vi "TraverseControl.vi"(0 "Mode":T6=enum."Read traverse position", 1 "Work in Tunnel Coordinates?":T3, 2 "Probe Support":T2=[{"Max"=15001.0, "Min"=12000.0}, {"Max"=1000.0, "Min"=-1000.0}, {"Max"=700.0, "Min"=0.0}] {"Min" format="%#.1f"; "Max" format="%#.1f"}, 3 "Model       Roll      Pitch       Yaw (deg)":sgl[](array[numeric]) format="%#.2f", 4 "Probe Volume":T2=[{"Max"=15.0, "Min"=-15.0}, {"Max"=250.0, "Min"=0.0}, {"Max"=15.0, "Min"=-15.0}] {"Min" format="%#.1f"; "Max" format="%#.1f"}, 5 "Position input XYZ":sgl[](array[numeric])=[0.0, 0.0, 0.0] format="%.2f", 6 "Route Checking?":bool, 7 "Entire Space":T2=[{"Max"=15001.0, "Min"=12000.0}, {"Max"=1000.0, "Min"=-1000.0}, {"Max"=700.0, "Min"=0.0}] {"Min" format="%#.1f"; "Max" format="%#.1f"}, 8 "Last Part of Move?":bool, 9 "Home":T1, 10 "Exclude Array":T4[](array[typedef]) {"Sizes"."Min" format="%#.1f"; "Sizes"."Max" format="%#.1f"}, 11 "Speed Factor":sgl=1.0 min=0.1 max=5 format="%.2f", 12 "Traverse Name":string, 13 "Backlash Compensation?":bool=TRUE, 15 "Trav_Coordinates New Pos dx;dy;dz":sgl[](array[numeric])=[0.0, 0.0, 0.0] format="%.2f", 16 "Trav_Coordinates Current Pos dx;dy;dz":sgl[](array[numeric])=[0.0, 0.0, 0.0] format="%.2f") -> (14 "Position Output XYZ":sgl[](array[numeric]) format="%.2f", 17 "Moved?":bool, 18 "Position Correct":bool, 19 "Error String":string)   [LabVIEW 2022 SP3]
uses:
  Anemometry/Anemometry Sub Vis/Gen Trav/Trav_mode.ctl
  Anemometry/Anemometry Sub Vis/Gen Trav/Route mapping/Exclude_cluster.ctl
  Anemometry/Anemometry Sub Vis/Gen Trav/Route mapping/Box_size.ctl
  Anemometry/Anemometry Sub Vis/Gen Trav/Route mapping/Exclusion_type.ctl
  Anemometry/Anemometry Sub Vis/Controls/Tunnel_Coordinates.ctl
  Anemometry/Anemometry Sub Vis/Controls/Home.ctl
  ~subVIs/GenericDriveCommand.ctl
  ADAM Client/Sub VIs/ADAM Controls/Update_scan_value.ctl
  Anemometry/Anemometry Sub Vis/Globals/Preference_global.vi
  Anemometry/Anemometry Sub Vis/Globals/Trav_pos_global.vi
  ~subVIs/DriveConfigGlobal.vi
  ~subVIs/Traverse Type.ctl
panel:
  out "Config the same?":bool[](array[boolean])
  out "Position Steps":sgl[][](array[numeric]) format="%.2f"
  out "Log File":path
  out "Achieved Pos In Eng units of all channels":sgl[](array[numeric]) format="%.2f"
  out "Pulses Positon all channels":sgl[](array[numeric])
  out "Counters Reset?":bool
  # "X                Y                   Z"
  # "X                           Y                          Z"
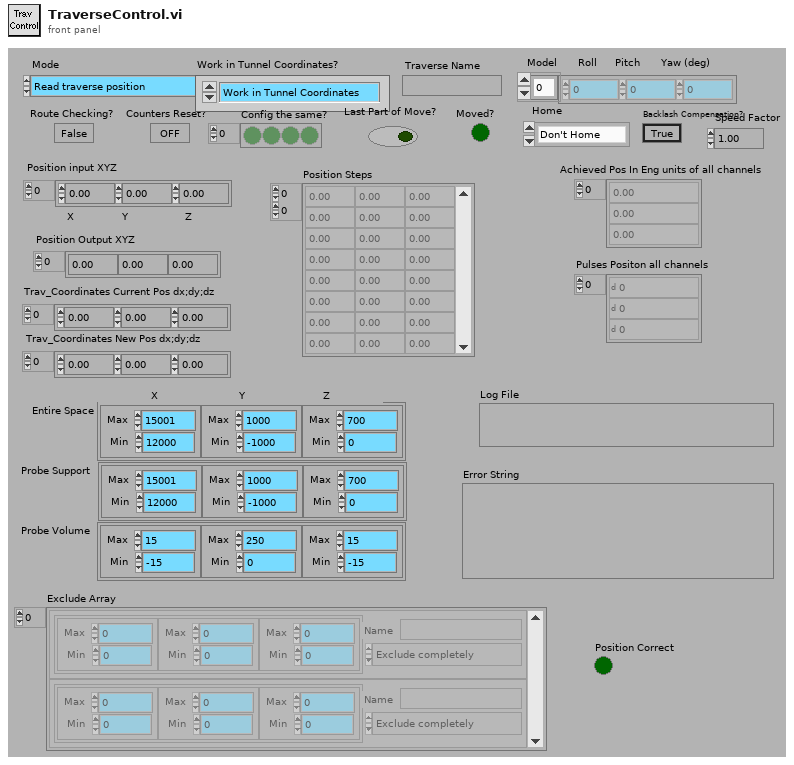
[diagram p1: front panel]
types:
  T1 = typedef "Home.ctl" = enum16{"Don't Home", "Home  +X", "Home  -X", "Home  +Y", "Home  -Y", "Home  +Z", "Home  -Z"}
  T2 = typedef "Box_size.ctl" = cluster{"Max":sgl, "Min":sgl}[]
  T3 = typedef "Tunnel_Coordinates.ctl" = enum16{"Work in Tunnel Coordinates", "Work in Model Coordinates"}
  T4 = typedef "Exclude_cluster.ctl" = cluster{"Sizes":T2, "Name":string, "Exclude Type":T5}
  T5 = typedef "Exclusion_type.ctl" = enum16{"Exclude completely", "Allow only vertical moves"}
  T6 = typedef "Trav_mode.ctl" = enum16{"Move traverse", "Read traverse position", "Teach Position"}
  T7 = typedef "Traverse Type.ctl" = enum16{"MCode", "Dynamixel"}
  T8 = typedef "GenericDriveCommand.ctl" = string
  T9 = enum16{"To Traverse Coordinates", "To User Coordinates"}
  T10 = typedef "DriveProperties.ctl" = cluster{"Channel Name":string, "Vel. Default":sgl, "Acc. Default":sgl, "Vel. Max":sgl, "Vel. Min":sgl, "Acc. Max":sgl, "Acc. Min":sgl, "Pulses/unit":sgl, "Address":u8, "Pulse Offset":i32, "Pos Tolerance":sgl, "Pulses/rev":sgl, "Backlash/Eng units":sgl, "Current Pos":sgl, "Ch Status":enum16{"Active", "Offline", "Simulate"}, "Port Name":string, "Axis Transform mode":string, "Metadata Ch Name":string, "Type":T7, "De Power Motor":enum16{"TRUE", "FALSE"}, "ConfigString":string}
  T11 = typedef "Update_scan_value.ctl" = cluster{"Channel Name":string, "New Value":dbl, "!Auto_Off":bool}
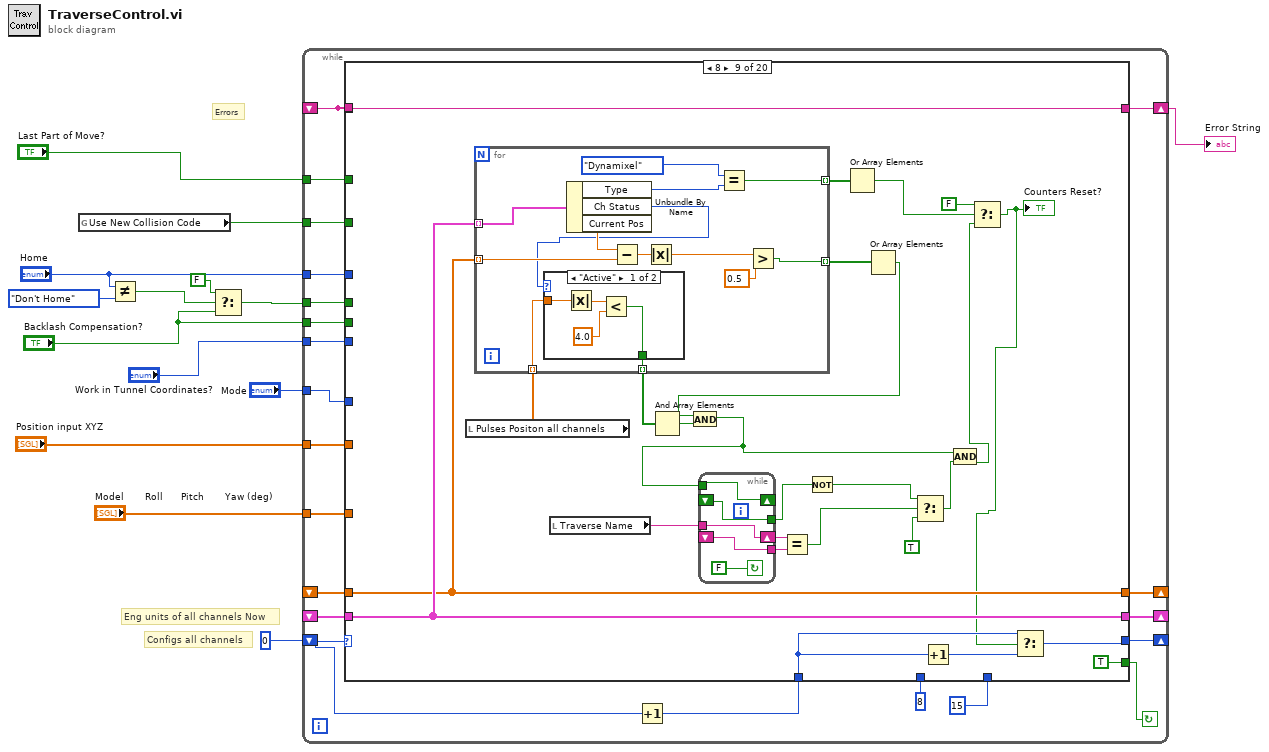
[diagram p0: block diagram]
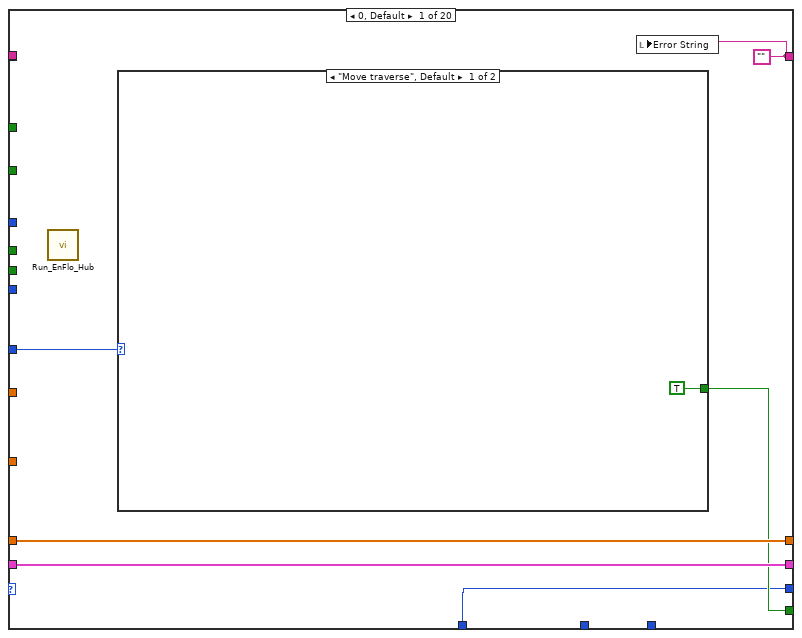
[diagram p2: hidden frame]
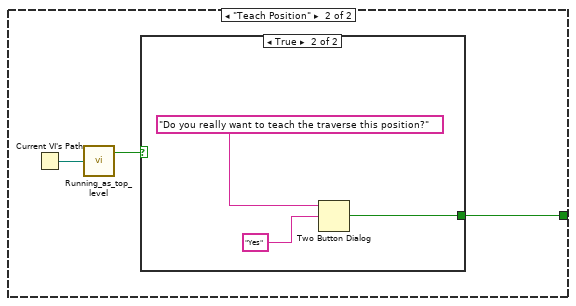
[diagram p3: hidden frame]
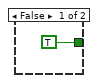
[diagram p4: hidden frame]
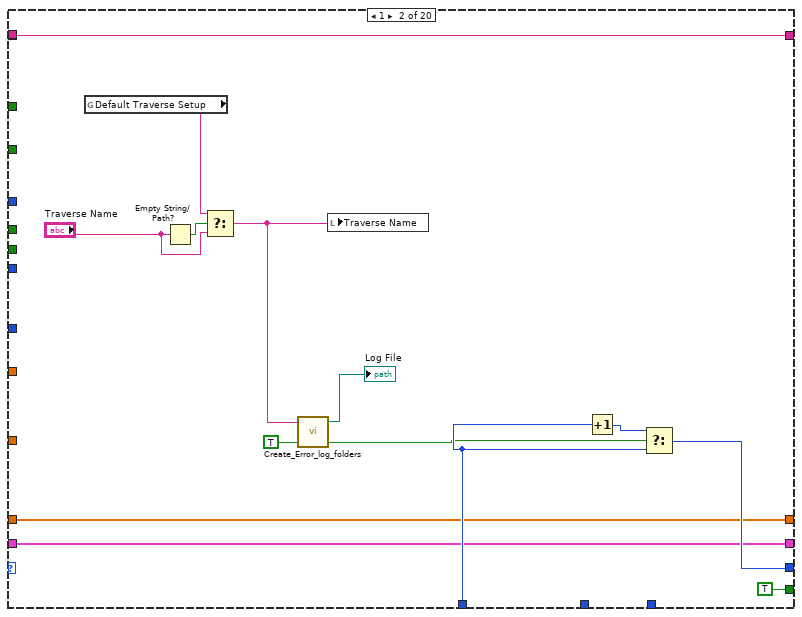
[diagram p5: hidden frame]
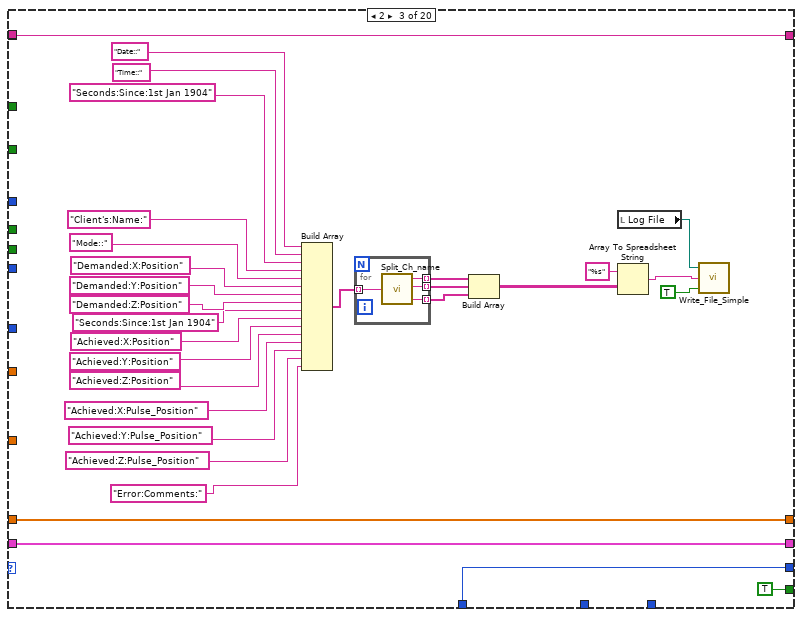
[diagram p6: hidden frame]
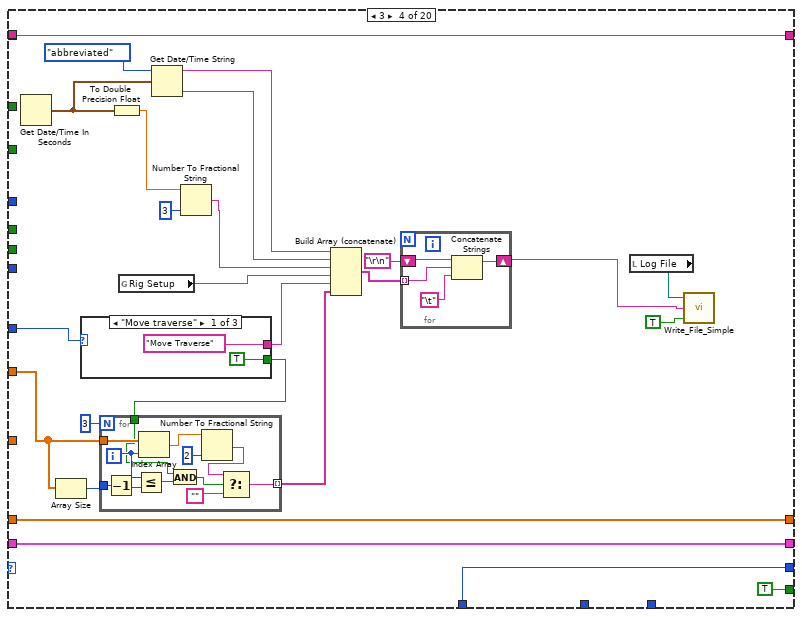
[diagram p7: hidden frame]
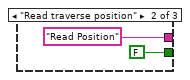
[diagram p8: hidden frame]
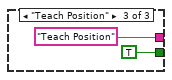
[diagram p9: hidden frame]
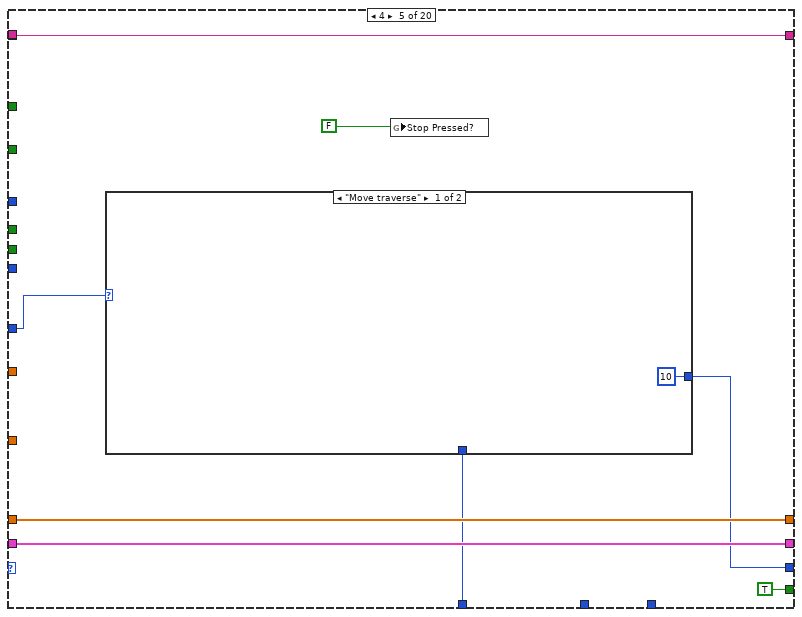
[diagram p10: hidden frame]
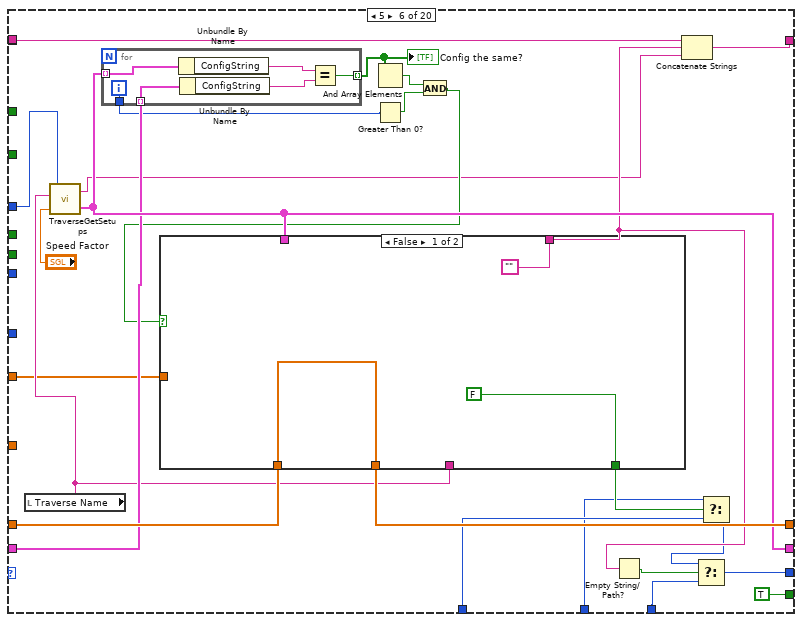
[diagram p12: hidden frame]
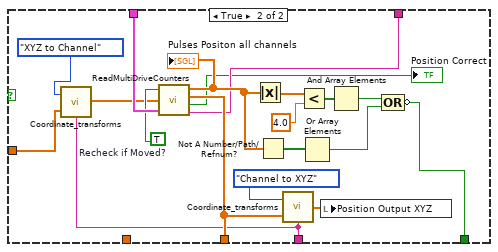
[diagram p13: hidden frame]
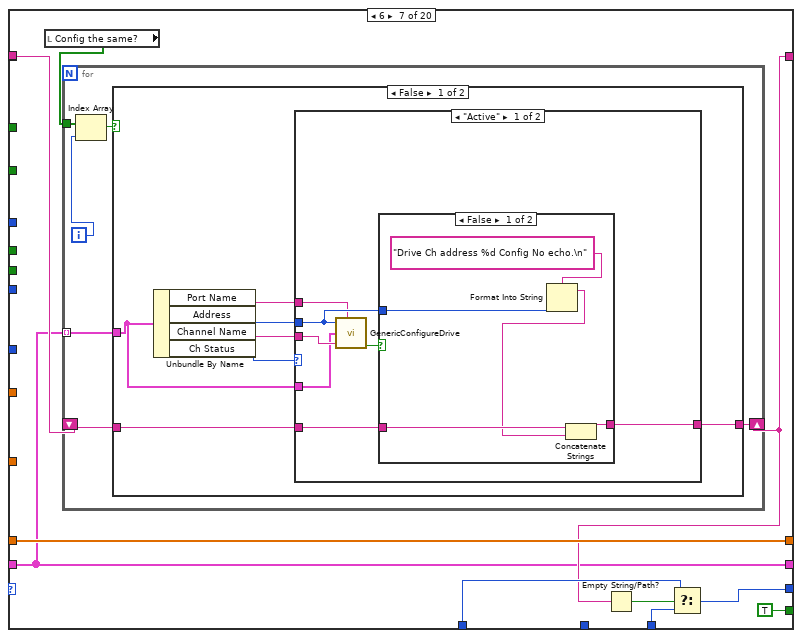
[diagram p14: hidden frame]
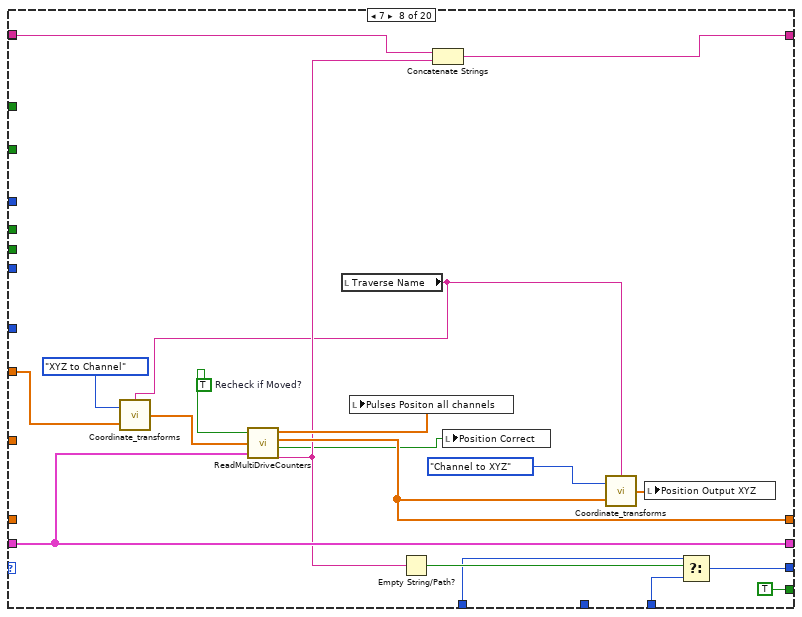
[diagram p18: hidden frame]
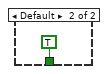
[diagram p19: hidden frame]
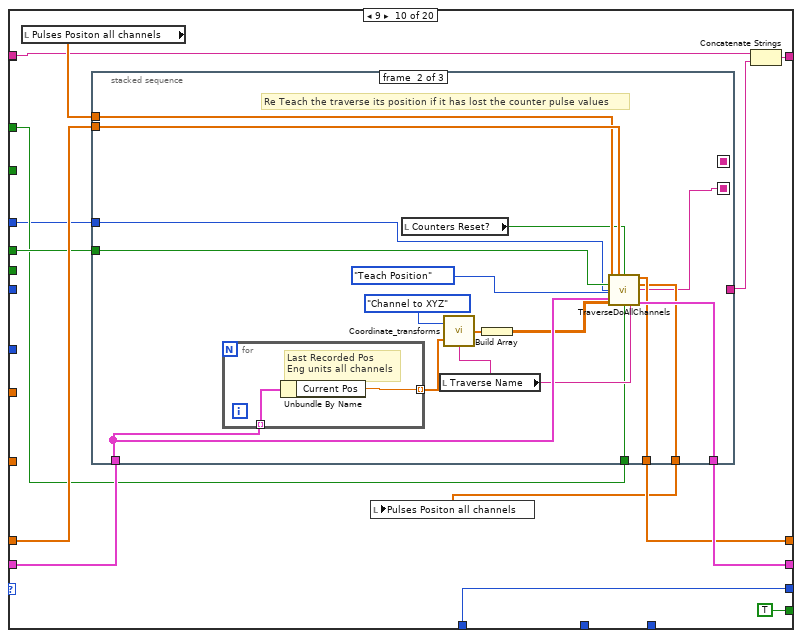
[diagram p20: hidden frame]
diagram:
  # "Errors"
  # "Eng units of all channels Now"
  # "Configs all channels"
  n1 = global read "Preference_global.vi" "Use New Collision Code"() -> (w3:bool)
  n2 = Not Equal?(x="Home", y=Home."Don't Home" ("Home")) -> (x != y?=w4:bool)
  n3 = Select(t=FALSE, s=w4, f="Backlash Compensation?") -> (s? t:f=w8:bool)
  n4 = while {
    tunnel: w8 -> [w22]
    tunnel: "Position input XYZ" -> [w26]
    shift-left: _ -> [w23]
    shift-right: [w27] -> w12
    shift-left: _ -> [w28]
    shift-right: [w29] -> _
    shift-left: _ -> [w17]
    shift-right: [w30] -> _
    shift-left: 0 -> [w33]
    shift-right: [w31] -> _
    tunnel: "Mode" -> [w35]
    tunnel: "Model       Roll      Pitch       Yaw (deg)" -> [w21]
    tunnel: "Work in Tunnel Coordinates?" -> [w20]
    tunnel: "Last Part of Move?" -> [w19]
    tunnel: "Home" -> [w18]
    tunnel: w3 -> [w16]
    tunnel: "Backlash Compensation?" -> [w15]
    stop <- w34 continue-if-true
    n5 = Increment(x=w33) -> (x+1=w32:i32)
    n6 = case shown="8" w33 {
      tunnel: w35 -> [w41 _ _ w115 w147 _ _ _ _ _ w380 _ w482 w495 _ _ _ w577 _ w633]
      tunnel: [w38 TRUE ("T button?") TRUE ("T button?") TRUE ("T button?") TRUE TRUE ("T button?") TRUE ("T button?") TRUE ("T button?") TRUE TRUE TRUE ("T button?") TRUE ("T button?") TRUE TRUE TRUE ("T button?") TRUE ("T button?") TRUE ("T button?") w579 TRUE FALSE] -> w34
      tunnel: w32 -> [w37 w62 w73 w120 w145 w176 w214 w253 w289 w318 w379 w403 w473 w497 w529 w546 w572 w576 w611 w640]
      tunnel: [w37 w60 w73 w120 w146 w159 w213 w251 w287 w318 w378 w404 w473 w496 w529 w544 w572 w575 w611 w640] -> w31
      tunnel: [w39 w57 w75 w122 w149 w174 w209 w264 w285 w327 w376 w406 w466 w494 w531 w555 w574 w582 w609 w638] -> w30
      tunnel: w17 -> [w39 w57 w75 w122 w149 w173 w209 w264 w285 w326 w376 w406 w480 w494 w531 w555 w574 w582 w609 w638]
      tunnel: [w40 w58 w74 w121 w150 w179 w217 w259 w284 w323 w375 w396 w474 w500 w530 w554 w573 w583 w612 w641] -> w29
      tunnel: w28 -> [w40 w58 w74 w121 w150 w178 w217 _ w284 w324 w375 w396 w469 w500 w530 w554 w573 w583 w612 w641]
      tunnel: [w36 w56 w71 w112 w151 w164 w210 w256 w286 w320 w381 w399 w476 w498 w527 w532 w570 w578 w605 w634] -> w27
      tunnel: w23 -> [_ w56 w71 w112 w151 w165 w211 w257 w286 w322 w381 _ w477 w498 w527 w532 w570 w581 w607 w636]
      tunnel: w26 -> [_ _ _ w109 _ w155 _ w249 _ _ w374 w398 _ _ _ _ _ _ w603 _]
      tunnel: 15 ("f") -> [_ _ _ _ _ w160 w212 w252 _ _ _ w401 _ _ _ _ _ _ _ _]
      tunnel: 8 ("t") -> [_ _ _ _ _ w175 _ _ _ _ _ _ _ _ _ _ _ _ _ _]
      tunnel: w23 -> [_ _ _ _ _ _ _ _ _ _ _ w402 _ _ _ _ _ _ _ _]
      tunnel: w22 -> [_ _ _ _ _ _ _ _ _ w317 _ _ w468 _ _ _ _ _ _ _]
      tunnel: w21 -> [_ _ _ _ _ _ _ _ _ _ _ w393 _ w491 _ _ _ _ w604 w631]
      tunnel: w20 -> [_ _ _ _ _ _ _ _ _ _ _ _ _ _ _ _ _ _ w601 w629]
      tunnel: w19 -> [_ _ _ _ _ _ _ _ _ w315 _ _ w464 w485 _ _ _ _ _ _]
      tunnel: w18 -> [_ _ _ _ _ w157 _ _ _ w314 _ _ w463 _ _ _ _ _ _ _]
      tunnel: w16 -> [_ _ _ _ _ _ _ _ _ _ _ w392 _ _ _ _ _ _ _ _]
      tunnel: w15 -> [_ _ _ _ _ _ _ _ _ _ _ _ _ w484 _ _ _ _ _ _]
      frame 0, Default {
        w36 = ""
        n7 = call "Run_EnFlo_Hub.vi"() -> ()  [unwired: 1 in, 7 out]
        n8 = case shown="\"Move traverse\", Default" w41 {
          tunnel: [TRUE ("T button?") w43] -> w38
          frame "Move traverse", Default {
          }
          frame "Teach Position" {
            n9 = Current VI's Path() -> (path=w45:path)
            n10 = call "Running_as_top_level.vi"("Vi path name"=w45) -> ("Top Level"=w44:bool)  [unwired: 1 out]
            n11 = case shown="True" w44 {
              tunnel: [TRUE ("T button?") w47] -> w43
              frame False {
              }
              frame True {
                n12 = Two Button Dialog(message="Do you really want to teach the traverse this position?", 2:"Yes" ("T button name (\"OK\")")) -> (T button?=w47:bool)  [unwired: 1 out]
              }
            }
          }
        }
        n13 = local write "Error String"(w36) -> ()
      }
      frame 1 {
        n14 = global read "Trav_pos_global.vi" "Default Traverse Setup"() -> (w54:string)
        n15 = Empty String/Path?(string/path="Traverse Name") -> (empty?=w52:bool)
        n16 = Select(t=w54, s=w52, f="Traverse Name") -> (s? t:f=w50:string)
        n17 = call "Create_Error_log_folders.vi"("Log Filename"=w50, "Per Day Log File?"=TRUE) -> ("Local Log File"=→"Log File":path, "exists?"=w55:bool)  [unwired: 4 in]
        n18 = local write "Traverse Name"(w50) -> ()
        n19 = Increment(x=w62) -> (x+1=w61:i32)
        n20 = Select(t=w61, s=w55, f=w62) -> (s? t:f=w60:i32)
      }
      frame 2 {
        n21 = Build Array("Date::", "Time::", "Seconds:Since:1st Jan 1904", "Client's:Name:", "Mode::", "Demanded:X:Position", "Demanded:Y:Position", "Demanded:Z:Position", "Seconds:Since:1st Jan 1904", "Achieved:X:Position", "Achieved:Y:Position", "Achieved:Z:Position", "Achieved:X:Pulse_Position", "Achieved:Y:Pulse_Position", "Achieved:Z:Pulse_Position", "Error:Comments:") -> (w78:string[])
        n22 = for {
          tunnel: w78 -> [w97] mode=indexing
          tunnel: [w96] -> w79 mode=indexing
          tunnel: [w95] -> w80 mode=indexing
          tunnel: [w94] -> w81 mode=indexing
          n23 = call "Split_Ch_name.vi"("Ch name"=w97) -> ("Top level"=w96:string, "Middle"=w95:string, "Low level"=w94:string)
        }
        n24 = Build Array(w79, w80, w81) -> (w76:string[][])
        n25 = local read "Log File"() -> (w68:path)
        n26 = Array To Spreadsheet String(array=w76, 3:"%s" ("format string")) -> (spreadsheet string=w69:string)  [unwired: 1 out]
        n27 = call "Write_File_Simple.vi"("append to file? (new file:F)"=TRUE, "character string"=w69, "file path"=w68) -> ()  [unwired: 2 out]
      }
      frame 3 {
        n28 = Get Date/Time In Seconds() -> (seconds since 1Jan1904=w102:timestamp)
        n29 = Array Size(array=w109) -> (size(s)=w110:i32)
        n30 = case shown="\"Move traverse\"" w115 {
          tunnel: ["Move Traverse" "Read Position" "Teach Position"] -> w116
          tunnel: [TRUE FALSE TRUE] -> w106
          frame "Move traverse" {
          }
          frame "Read traverse position" {
          }
          frame "Teach Position" {
          }
        }
        n31 = for {
          N: 3 -> [_]
          tunnel: w109 -> [w134]
          tunnel: w110 -> [w131]
          tunnel: [w127] -> w107 mode=indexing
          tunnel: w106 -> [w123]
          i -> [w129]
          n32 = Decrement(x=w131) -> (x-1=w130:i32)
          n33 = Less Or Equal?(x=w129, y=w130) -> (x <= y?=w125:bool)
          n34 = Index Array(array=w134, index=w129) -> (element=w133:sgl)
          n35 = And(x=w123, y=w125) -> (x .and. y?=w124:bool)
          n36 = Number To Fractional String(number=w133, precision (6)=i16 2) -> (F-format string=w128:string)  [unwired: 2 out]
          n37 = Select(t=w128, s=w124, f="") -> (s? t:f=w127:string)
        }
        n38 = To Double Precision Float(number=w102) -> (double precision float=w101:dbl)
        n39 = global read "Preference_global.vi" "Rig Setup"() -> (w98:string)
        n40 = Get Date/Time String(date format (0)=enum16{"short", "long", "abbreviated"}."abbreviated", seconds (now)=w102) -> (date string=w118:string, time string=w117:string)  [unwired: 1 out]
        n41 = Number To Fractional String(number=w101, precision (6)=i16 3) -> (F-format string=w99:string)  [unwired: 2 out]
        n42 = Build Array (concatenate)(w118, w117, w99, w98, w116, w107) -> (w113:string[])
        n43 = for {
          shift-right: [w137] -> w103
          shift-left: "\r\n" -> [w138]
          tunnel: w113 -> [w136] mode=indexing
          n44 = Concatenate Strings(w138, w136, "\t") -> (w137:string)
        }
        n45 = local read "Log File"() -> (w104:path)
        n46 = call "Write_File_Simple.vi"("append to file? (new file:F)"=TRUE, "character string"=w103, "file path"=w104) -> ()  [unwired: 2 out]
      }
      frame 4 {
        n47 = case shown="\"Move traverse\"" w147 {
          tunnel: [10 w154] -> w146
          tunnel: w145 -> [_ w154]
          frame "Move traverse" {
          }
          frame "Read traverse position", Default {
          }
        }
        n48 = global write "DriveConfigGlobal.vi" "Stop Pressed?"(FALSE) -> ()
      }
      frame 5 {
        n49 = local read "Traverse Name"() -> (w167:string)
        n50 = call "TraverseGetSetups.vi"("Speed Factor"="Speed Factor", "Traverse Name"=w167, "Home"=w157) -> ("Channel Properties Out"=w174:T10[], "Error String"=w156:string)
        n51 = for {
          tunnel: w174 -> [w185] mode=indexing
          tunnel: w173 -> [w184] mode=indexing
          tunnel: [w181] -> w172 mode=indexing
          tunnel: [w180] -> w171
          i -> [w180]
          n52 = Unbundle By Name(w185) -> ("ConfigString"=w183:string)
          n53 = Unbundle By Name(w184) -> ("ConfigString"=w182:string)
          n54 = Equal?(x=w183, y=w182) -> (x = y?=w181:bool)
        }
        "Config the same?" <- w172
        n55 = And Array Elements(Boolean array=w172) -> (logical AND=w169:bool)
        n56 = Greater Than 0?(x=w171) -> (x > 0?=w170:bool)
        n57 = And(x=w169, y=w170) -> (x .and. y?=w168:bool)
        n58 = case shown="False" w168 {
          tunnel: w174 -> [_ w207]
          tunnel: [w188 w197] -> w179
          tunnel: w178 -> [w188 _]
          tunnel: [FALSE w199] -> w177
          tunnel: w167 -> [_ w191]
          tunnel: ["" w194] -> w163
          tunnel: w155 -> [_ w193]
          frame False {
          }
          frame True {
            w195 = TRUE  # Recheck if Moved?
            n59 = call "Coordinate_transforms.vi"("Traverse Name"=w191, "Input"=w193, "Mode"=enum16{"XYZ to Channel", "Channel to XYZ"}."XYZ to Channel") -> ("Output"=w190:sgl[])
            n60 = call "ReadMultiDriveCounters.vi"("Recheck if Moved?"=w195, "Position input XYZ"=w190, "Channel Properties"=w207) -> ("Pulses"=w202:sgl[], "Eng units"=w197:sgl[], "Position Correct"=→"Position Correct":bool, "Error String"=w194:string)
            "Pulses Positon all channels" <- w202
            n61 = Absolute Value(x=w202) -> (abs(x)=w206:sgl[])
            n62 = Not A Number/Path/Refnum?(number/path/refnum=w202) -> (NaN/Path/Refnum?=w201:bool[])
            n63 = call "Coordinate_transforms.vi"("Traverse Name"=w191, "Input"=w197, "Mode"=enum16{"XYZ to Channel", "Channel to XYZ"}."Channel to XYZ") -> ("Output"=w196:sgl[])
            n64 = Less?(x=w206, y=sgl 4.0 ("Achieved Position")) -> (x < y?=w204:bool[])
            n65 = Or Array Elements(Boolean array=w201) -> (logical OR=w200:bool)
            n66 = local write "Position Output XYZ"(w196) -> ()
            n67 = And Array Elements(Boolean array=w204) -> (logical AND=w203:bool)
            n68 = Compound Arithmetic op=OR(w203, w200) -> (invert w199:bool)
          }
        }
        n69 = Empty String/Path?(string/path=w163) -> (empty?=w162:bool)
        n70 = Concatenate Strings(w165, w163, w156) -> (w164:string)
        n71 = Select(t=w175, s=w177, f=w176) -> (s? t:f=w161:i32)
        n72 = Select(t=w161, s=w162, f=w160) -> (s? t:f=w159:i32)
      }
      frame 6 {
        n73 = local read "Config the same?"() -> (w208:bool[])
        n74 = for {
          tunnel: w209 -> [w223] mode=indexing
          shift-right: [w221] -> w210
          shift-left: w211 -> [w222]
          tunnel: w208 -> [w219]
          i -> [w220]
          n75 = Index Array(array=w219, index=w220) -> (element=w218:bool)
          n76 = case shown="False" w218 {
            tunnel: w223 -> [w224 _]
            tunnel: w222 -> [w226 w245]
            tunnel: [w225 w245] -> w221
            frame False {
              n77 = Unbundle By Name(w224) -> ("Port Name"=w227:string, "Address"=w230:u8, "Channel Name"=w229:string, "Ch Status"=w228:enum16{"Active", "Offline", "Simulate"})
              n78 = case shown="\"Active\"" w228 {
                tunnel: w230 -> [w236 _]
                tunnel: w229 -> [w237 _]
                tunnel: w227 -> [w235 _]
                tunnel: w226 -> [w233 w244]
                tunnel: [w232 w244] -> w225
                tunnel: w224 -> [w231 _]
                frame "Active" {
                  n79 = call "GenericConfigureDrive.vi"("Address"=w236, "Port Name"=w235, "Channel Properties In"=w231, "Channel Name"=w237) -> ("Good Echo"=w234:bool)  [unwired: 4 out]
                  n80 = case shown="False" w234 {
                    tunnel: w236 -> [w242 _]
                    tunnel: w233 -> [w240 w243]
                    tunnel: [w239 w243] -> w232
                    frame False {
                      n81 = Format Into String(format string="Drive Ch address %d Config No echo.\n" ("Format String"), w242) -> (resulting string=w238:string)  [unwired: 2 in, 1 out]
                      n82 = Concatenate Strings(w240, w238) -> (w239:string)
                    }
                    frame True {
                    }
                  }
                }
                frame "Offline", Default {
                }
              }
            }
            frame True {
            }
          }
        }
        n83 = Empty String/Path?(string/path=w210) -> (empty?=w215:bool)
        n84 = Select(t=w214, s=w215, f=w212) -> (s? t:f=w213:i32)
      }
      frame 7 {
        w258 = TRUE  # Recheck if Moved?
        n85 = local read "Traverse Name"() -> (w247:string)
        n86 = call "Coordinate_transforms.vi"("Traverse Name"=w247, "Input"=w249, "Mode"=enum16{"XYZ to Channel", "Channel to XYZ"}."XYZ to Channel") -> ("Output"=w248:sgl[])
        n87 = call "ReadMultiDriveCounters.vi"("Recheck if Moved?"=w258, "Position input XYZ"=w248, "Channel Properties"=w264) -> ("Pulses"=w262:sgl[], "Eng units"=w259:sgl[], "Position Correct"=w246:bool, "Error String"=w254:string)
        n88 = local write "Pulses Positon all channels"(w262) -> ()
        n89 = Empty String/Path?(string/path=w254) -> (empty?=w255:bool)
        n90 = Concatenate Strings(w257, w254) -> (w256:string)
        n91 = local write "Position Correct"(w246) -> ()
        n92 = call "Coordinate_transforms.vi"("Traverse Name"=w247, "Input"=w259, "Mode"=enum16{"XYZ to Channel", "Channel to XYZ"}."Channel to XYZ") -> ("Output"=w260:sgl[])
        n93 = local write "Position Output XYZ"(w260) -> ()
        n94 = Select(t=w253, s=w255, f=w252) -> (s? t:f=w251:i32)
      }
      frame 8 {
        n95 = local read "Pulses Positon all channels"() -> (w272:sgl[])
        n96 = for {
          tunnel: w285 -> [w308] mode=indexing
          tunnel: w284 -> [w306] mode=indexing
          tunnel: [w302] -> w283 mode=indexing
          tunnel: w272 -> [w301] mode=indexing
          tunnel: [w299] -> w271 mode=indexing
          tunnel: [w297] -> w269 mode=indexing
          n97 = Unbundle By Name(w308) -> ("Type"=w298:T7, "Ch Status"=w300:enum16{"Active", "Offline", "Simulate"}, "Current Pos"=w307:sgl)
          n98 = case shown="\"Active\"" w300 {
            tunnel: w301 -> [w311 _]
            tunnel: [w309 TRUE] -> w299
            frame "Active" {
              n99 = Absolute Value(x=w311) -> (abs(x)=w312:sgl)
              n100 = Less?(x=w312, y=4.0 ("Achieved Position")) -> (x < y?=w309:bool)
            }
            frame Default {
            }
          }
          n101 = Subtract(x=w307, y=w306) -> (x-y=w305:sgl)
          n102 = Absolute Value(x=w305) -> (abs(x)=w304:sgl)
          n103 = Equal?(x=Traverse_Type."Dynamixel" ("Type"), y=w298) -> (x = y?=w297:bool)
          n104 = Greater?(x=w304, y=0.5) -> (0:w302:bool)
        }
        n105 = local read "Traverse Name"() -> (w273:string)
        n106 = And Array Elements(Boolean array=w271) -> (logical AND=w270:bool)
        n107 = Or Array Elements(Boolean array=w269) -> (logical OR=w268:bool)
        n108 = Or Array Elements(Boolean array=w283) -> (logical OR=w282:bool)
        n109 = And(x=w282, y=w270) -> (x .and. y?=w281:bool)
        n110 = while {
          tunnel: [w294] -> w275
          tunnel: w281 -> [w295]
          shift-left: _ -> [w294]
          shift-right: [w295] -> _
          shift-right: [w292] -> w280
          shift-left: _ -> [w291]
          tunnel: w273 -> [w292]
          tunnel: [w291] -> w279
          stop <- FALSE continue-if-true
        }
        n111 = Equal?(x=w280, y=w279) -> (x = y?=w278:bool)
        n112 = Not(x=w275) -> (.not. x?=w274:bool)
        n113 = Select(t=w274, s=w278, f=TRUE) -> (s? t:f=w277:bool)
        n114 = Increment(x=w289) -> (x+1=w288:i32)
        n115 = Compound Arithmetic op=AND(w281, w277) -> (w267:bool)
        n116 = Select(t=FALSE, s=w268, f=w267) -> (s? t:f=w265:bool)
        "Counters Reset?" <- w265
        n117 = Select(t=w289, s=w265, f=w288) -> (s? t:f=w287:i32)
      }
      frame 9 {
        n118 = local read "Pulses Positon all channels"() -> (w325:sgl[])
        n119 = stacked-sequence {
          seq-local: [w328 _ _] -> [_ _ w353]
          seq-local: [_ w332 _] -> [_ _ w352]
          tunnel: w325 -> [_ w341 w355]
          tunnel: [_ w348 _] -> w327
          tunnel: w324 -> [_ w347 _]
          tunnel: [_ w346 _] -> w323
          tunnel: w326 -> [_ w343 w356]
          tunnel: [_ _ w351] -> w321
          tunnel: w317 -> [_ w337 _]
          tunnel: [_ w335 _] -> w316
          tunnel: w315 -> [w329 w334 _]
          tunnel: w314 -> [_ w333 _]
          frame #0 {
            n120 = case shown="True" w329 {
              tunnel: ["" w331] -> w328
              frame False {
              }
              frame True {
                n121 = call "Shut_down_all_Axis.vi"() -> ("Error String"=w331:string)  [unwired: 1 in]
              }
            }
          }
          frame #1 {
            # "Re Teach the traverse its position if it has lost the counter pulse values"
            n122 = for {
              tunnel: [w350] -> w342 mode=indexing
              tunnel: w343 -> [w349] mode=indexing
              # "Last Recorded Pos\nEng units all channels"
              n123 = Unbundle By Name(w349) -> ("Current Pos"=w350:sgl)
            }
            n124 = local read "Counters Reset?"() -> (w339:bool)
            n125 = local read "Traverse Name"() -> (w338:string)
            n126 = call "Coordinate_transforms.vi"("Traverse Name"=w338, "Input"=w342, "Mode"=enum16{"XYZ to Channel", "Channel to XYZ"}."Channel to XYZ") -> ("Output"=w344:sgl[])
            n127 = Build Array(w344) -> (w336:sgl[][])
            n128 = call "TraverseDoAllChannels.vi"("Current Pulses positions for all channels"=w341, "Current Pos In Eng units of all channels"=w347, "Counters Reset?"=w339, "Backlash Compensation?"=w337, "Home"=w333, "Mode"=Trav_mode."Teach Position", "Position Steps"=w336, "Channel Properties"=w343, "Last Part of Move?"=w334, "Traverse Name"=w338) -> ("Achieved Pos In Eng units of all channels"=w346:sgl[], "Current Pulses positions for all channels Out"=w335:sgl[], "Error String"=w332:string, "Channel Properties Out"=w348:T10[])  [unwired: 1 in, 1 out]
          }
          frame #2 {
            n129 = for {
              tunnel: w356 -> [w364] mode=indexing
              tunnel: w355 -> [w363] mode=indexing
              tunnel: [w357] -> w354 mode=indexing
              n130 = Unbundle By Name(w364) -> ("Ch Status"=w362:enum16{"Active", "Offline", "Simulate"}, "Port Name"=w361:string, "Type"=w360:T7, "Address"=w359:u8, "Channel Name"=w358:string)
              n131 = case shown="\"Active\"" w362 {
                tunnel: w363 -> [w371 _]
                tunnel: w361 -> [w370 _]
                tunnel: w360 -> [w369 _]
                tunnel: w359 -> [w368 _]
                tunnel: w358 -> [w367 _]
                tunnel: [w365 ""] -> w357
                frame "Active" {
                  n132 = call "GenericDriveIO.vi"("GenericDriveCommand"=T8 "PositionSetTarget", "Channel Name"=w367, "Numeric Value"=w371, "Address"=w368, "Type"=w369, "Port Name"=w370) -> ("Error Description"=w365:string)  [unwired: 1 in, 4 out]
                }
                frame "Offline", Default {
                }
              }
            }
            n133 = Concatenate Strings(w352, w353, w354) -> (w351:string)
          }
        }
        n134 = local write "Pulses Positon all channels"(w316) -> ()
        n135 = Concatenate Strings(w322, w321) -> (w320:string)
      }
      frame 10 {
        n136 = Build Array(w374) -> (w373:sgl[][])
        n137 = local write "Position Steps"(w373) -> ()
        n138 = case shown="\"Read traverse position\", Default" w380 {
          tunnel: w379 -> [w382 w389]
          tunnel: [w384 w388] -> w378
          frame "Move traverse" {
            n139 = Increment(x=w382) -> (x+1=w383:i32)
            n140 = case shown="True" "Route Checking?" {
              tunnel: [w386 w387] -> w384
              tunnel: w383 -> [w386 _]
              tunnel: w382 -> [_ w387]
              frame False {
              }
              frame True {
              }
            }
          }
          frame "Read traverse position", Default {
            n141 = Increment(x=w389) -> (x+1=w388:i32)
          }
        }
      }
      frame 11 {
        n142 = local read "Traverse Name"() -> (w397:string)
        n143 = case shown="True" w392 {
          tunnel: w398 -> [w412 w452]
          tunnel: w397 -> [w427 w455]
          tunnel: w396 -> [w426 w457]
          tunnel: [w423 w447] -> w395
          tunnel: [w422 w453] -> w394
          tunnel: w393 -> [w417 w456]
          tunnel: "Trav_Coordinates New Pos dx;dy;dz" -> [w408 w445]
          tunnel: "Trav_Coordinates Current Pos dx;dy;dz" -> [w407 w446]
          frame False {
            w421 = 0.1  # Reduce by
            w425 = TRUE  # Full Check
            n144 = for {
              tunnel: "Probe Volume" -> [w437] mode=indexing
              tunnel: [w436] -> w420 mode=indexing
              tunnel: w421 -> [w431]
              n145 = Unbundle By Name(w437) -> ("Max"=w435:sgl, "Min"=w433:sgl)
              n146 = Subtract(x=w435, y=w431) -> (x-y=w434:dbl)
              n147 = Add(x=w431, y=w433) -> (x+y=w432:dbl)
              n148 = Bundle By Name(cluster=w437, "Max"=w434, "Min"=w432) -> (w436:cluster{"Max":sgl, "Min":sgl})
            }
            n149 = Subtract(x=w412, y=w408) -> (x-y=w411:sgl[])
            n150 = call "Coordinate_transforms.vi"("Traverse Name"=w427, "Input"=w426, "Mode"=enum16{"XYZ to Channel", "Channel to XYZ"}."Channel to XYZ") -> ("Output"=w410:sgl[])
            n151 = Subtract(x=w410, y=w407) -> (x-y=w409:sgl[])
            n152 = call "Coordinate_rotation.vi"("Roll-Pitch-Yaw"=w417, "Input Position"=w411, "Mode"=T9."To User Coordinates") -> ("Output Position"=w429:sgl[])  [unwired: 2 in, 1 out]
            n153 = call "Coordinate_rotation.vi"("Roll-Pitch-Yaw"=w417, "Input Position"=w409, "Mode"=T9."To User Coordinates") -> ("Output Position"=w418:sgl[])  [unwired: 2 in, 1 out]
            n154 = call "Check_Traverse_move.vi"("Current position"=w418, "Traverse Name"=w427, "Full Check"=w425, "New Position"=w429, "Model       Roll      Pitch       Yaw (deg)"=w417, "Probe Volume"=w420, "Entire Space"="Entire Space", "Exclude Array"="Exclude Array", "Probe Support"="Probe Support") -> ("Steps"=w424:sgl[][], "Error Comments"=w422:string)  [unwired: 5 out]
            n155 = for {
              tunnel: w424 -> [w442] mode=indexing
              tunnel: [w439] -> w423 mode=indexing
              tunnel: w417 -> [w441]
              tunnel: w408 -> [w438]
              n156 = call "Coordinate_rotation.vi"("Roll-Pitch-Yaw"=w441, "Input Position"=w442, "Mode"=T9."To Traverse Coordinates") -> ("Output Position"=w440:sgl[])  [unwired: 2 in, 1 out]
              n157 = Add(x=w440, y=w438) -> (x+y=w439:sgl[])
            }
          }
          frame True {
            w454 = TRUE  # Full Check
            n158 = Subtract(x=w452, y=w445) -> (x-y=w451:sgl[])
            n159 = call "Coordinate_transforms.vi"("Traverse Name"=w455, "Input"=w457, "Mode"=enum16{"XYZ to Channel", "Channel to XYZ"}."Channel to XYZ") -> ("Output"=w450:sgl[])
            n160 = Subtract(x=w450, y=w446) -> (x-y=w449:sgl[])
            n161 = call "Check_Traverse_move_PN.vi"("Current position"=w449, "Traverse Name"=w455, "Full Check"=w454, "New Position"=w451, "Model       Roll      Pitch       Yaw (deg)"=w456, "Traverse Active Parts"=cluster{"X":bool, "XY":bool, "XYZ":bool} {"X"=TRUE, "XY"=TRUE, "XYZ"=TRUE}) -> ("Steps"=w448:sgl[][], "Error Comments"=w453:string)  [unwired: 7 in, 1 out]
            n162 = for {
              tunnel: w445 -> [w461]
              tunnel: w448 -> [w460] mode=indexing
              tunnel: [w459] -> w447 mode=indexing
              n163 = Add(x=w460, y=w461) -> (x+y=w459:sgl[])
            }
          }
        }
        "Position Steps" <- w395
        n164 = Empty String/Path?(string/path=w394) -> (empty?=w400:bool)
        n165 = Select(t=w403, s=w400, f=w401) -> (s? t:f=w404:i32)
        n166 = Concatenate Strings(w402, w394) -> (w399:string)
      }
      frame 12 {
        w471 = FALSE  # Counters Reset?
        n167 = local read "Pulses Positon all channels"() -> (w481:sgl[])
        n168 = local read "Traverse Name"() -> (w470:string)
        n169 = local read "Position Steps"() -> (w467:sgl[][])
        n170 = call "TraverseDoAllChannels.vi"("Current Pulses positions for all channels"=w481, "Current Pos In Eng units of all channels"=w469, "Counters Reset?"=w471, "Backlash Compensation?"=w468, "Home"=w463, "Mode"=w482, "Position Steps"=w467, "Channel Properties"=w480, "Last Part of Move?"=w464, "Traverse Name"=w470) -> ("Achieved Pos In Eng units of all channels"=w474:sgl[], "Current Pulses positions for all channels Out"=w465:sgl[], "Moved?"=→"Moved?":bool, "Error String"=w475:string, "Channel Properties Out"=w466:T10[])  [unwired: 1 in]
        "Achieved Pos In Eng units of all channels" <- w474
        n171 = call "Coordinate_transforms.vi"("Traverse Name"=w470, "Input"=w474, "Mode"=enum16{"XYZ to Channel", "Channel to XYZ"}."Channel to XYZ") -> ("Output"=→"Position Output XYZ":sgl[])
        n172 = local write "Pulses Positon all channels"(w465) -> ()
        n173 = Concatenate Strings(w477, w475) -> (w476:string)
      }
      frame 13 {
        w488 = T11 {"Channel Name"="", "New Value"=0.0, "!Auto_Off"=FALSE} ("Update Scan Value Cluster")
        n174 = global read "Trav_pos_global.vi" "ADAM Channels in Model Coordinates"() -> (w489:string[])
        n175 = Not And(1:w484, 2:w485) -> (0:w483:bool)
        n176 = case shown="True" w485 {
          frame False {
          }
          frame True {
            n177 = global write "DriveConfigGlobal.vi" "Run Emergency stop loop"(FALSE ("Run Emergency stop loop")) -> ()
          }
        }
        n178 = local read "Position Output XYZ"() -> (w493:sgl[])
        n179 = case shown="\"Read traverse position\"" w495 {
          tunnel: w493 -> [_ w525 _]
          frame "Move traverse" {
          }
          frame "Read traverse position" {
            n180 = local write "Position input XYZ"(w525) -> ()
          }
          frame "Teach Position" {
            n181 = local write "Mode"(Trav_mode."Teach Position" ("Mode")) -> ()
          }
        }
        n182 = for {
          tunnel: w494 -> [w524] mode=indexing
          tunnel: w488 -> [w523]
          tunnel: w493 -> [w521] mode=indexing
          tunnel: [w520] -> w487 mode=indexing if=w518
          n183 = Unbundle By Name(w524) -> ("Metadata Ch Name"=w522:string)
          n184 = Empty String/Path?(string/path=w522) -> (empty?=w519:bool)
          n185 = Bundle By Name(cluster=w523, "Channel Name"=w522, "New Value"=w521) -> (w520:T11)
          n186 = Not(x=w519) -> (.not. x?=w518:bool)
        }
        n187 = Concatenate Strings(w489) -> (w492:string)
        n188 = Empty String/Path?(string/path=w492) -> (empty?=w490:bool)
        n189 = case shown="True" w490 {
          tunnel: w491 -> [w508 _]
          tunnel: w489 -> [w505 _]
          tunnel: w488 -> [w504 _]
          tunnel: w487 -> [w502 w516]
          tunnel: [w501 w516] -> w486
          frame False {
            n190 = local read "Position Output XYZ"() -> (w507:sgl[])
            n191 = call "Coordinate_rotation.vi"("Roll-Pitch-Yaw"=w508, "Input Position"=w507, "Mode"=T9."To User Coordinates") -> ("Output Position"=w506:sgl[])  [unwired: 2 in, 1 out]
            n192 = for {
              tunnel: w506 -> [w515] mode=indexing
              tunnel: w505 -> [w513] mode=indexing
              tunnel: w504 -> [w514]
              tunnel: [w511] -> w503 mode=indexing if=w510
              n193 = Bundle By Name(cluster=w514, "Channel Name"=w513, "New Value"=w515) -> (w511:T11)
              n194 = Empty String/Path?(string/path=w513) -> (empty?=w512:bool)
              n195 = Not(x=w512) -> (.not. x?=w510:bool)
            }
            n196 = Build Array (concatenate)(w502, w503) -> (w501:T11[])
          }
          frame True {
          }
        }
        n197 = Increment(x=w497) -> (x+1=w496:i32)
        n198 = call "Update_Current_Value_client.vi"("Don't Bother with check?"=w483, "Update array in"=w486) -> ()
      }
      frame 14 {
      }
      frame 15 {
        n199 = local read "Pulses Positon all channels"() -> (w536:sgl[])
        n200 = local read "Position Output XYZ"() -> (w535:sgl[])
        n201 = Get Date/Time In Seconds() -> (seconds since 1Jan1904=w543:timestamp)
        n202 = To Double Precision Float(number=w543) -> (double precision float=w538:dbl)
        n203 = Number To Fractional String(number=w538, precision (6)=i16 3) -> (F-format string=w537:string)  [unwired: 2 out]
        n204 = call "Truncate_Excessive_Strings.vi"("String"=w532) -> ("Truncated String"=w533:string)  [unwired: 2 in]
        n205 = Build Array (concatenate)(w535, w536) -> (w534:sgl[])
        n206 = Array Size(array=w534) -> (size(s)=w549:i32)
        n207 = for {
          N: 6 -> [_]
          tunnel: w534 -> [w569]
          tunnel: w549 -> [w566]
          tunnel: [w561] -> w548 mode=indexing
          i -> [w564]
          n208 = Decrement(x=w566) -> (x-1=w565:i32)
          n209 = Less Or Equal?(x=w564, y=w565) -> (x <= y?=w563:bool)
          n210 = Index Array(array=w569, index=w564) -> (element=w568:sgl)
          n211 = Number To Fractional String(number=w568, precision (6)=i16 2) -> (F-format string=w562:string)  [unwired: 2 out]
          n212 = Select(t=w562, s=w563, f="") -> (s? t:f=w561:string)
        }
        n213 = Build Array (concatenate)(w537, w548, w533) -> (w551:string[])
        n214 = local read "Route Checking?"() -> (w547:bool)
        n215 = for {
          shift-right: [w558] -> w540
          shift-left: "" -> [w559]
          tunnel: w551 -> [w557] mode=indexing
          n216 = Concatenate Strings(w559, w557, "\t") -> (w558:string)
        }
        n217 = Increment(x=w546) -> (x+1=w545:i32)
        n218 = local read "Log File"() -> (w541:path)
        n219 = Select(t=w545, s=w547, f=w546) -> (s? t:f=w544:i32)
        n220 = call "Write_File_Simple.vi"("append to file? (new file:F)"=TRUE, "character string"=w540, "file path"=w541) -> ()  [unwired: 2 out]
      }
      frame 16 {
      }
      frame 17 {
        n221 = local read "Position Output XYZ"() -> (w584:sgl[])
        n222 = local read "Counters Reset?"() -> (w585:bool)
        n223 = Index Array(array=w584, index=2) -> (element=w590:sgl)
        n224 = Index Array(array=w584, index=0) -> (element=w592:sgl)
        n225 = Index Array(array=w584, index=1) -> (element=w591:sgl)
        n226 = Format Into String(format string="X= %.2f\tY= %.2f\tZ= %.2f" ("Format String"), w592, w591, w590) -> (resulting string=w593:string)  [unwired: 2 in, 1 out]
        n227 = case shown="\"Read traverse position\"" w577 {
          tunnel: w576 -> [w597 w599]
          tunnel: [w597 w598] -> w575
          frame "Move traverse", Default {
          }
          frame "Read traverse position" {
            n228 = Increment(x=w599) -> (x+1=w598:i32)
          }
        }
        n229 = Select(t="\nThe traverse was probably powered down since the last move. Its position has now been retaught and now all should be well.", s=w585, f="") -> (s? t:f=w586:string)
        n230 = call "Write_out_serial_log.vi"("Header message"=w593) -> ()
        n231 = Concatenate Strings(w581, w586) -> (w578:string)
        n232 = Empty String/Path?(string/path=w578) -> (empty?=w580:bool)
        n233 = Not(x=w580) -> (.not. x?=w579:bool)
      }
      frame 18 {
        # "Add demanded position"
        n234 = case shown="\"Work in Model Coordinates\"" w601 {
          tunnel: w604 -> [_ w619]
          tunnel: w603 -> [w614 w618]
          tunnel: [w614 w616] -> w602
          tunnel: [" (Tunnel Coordinates)" " (Model Coordinates)"] -> w600
          frame "Work in Tunnel Coordinates" {
          }
          frame "Work in Model Coordinates" {
            n235 = call "Coordinate_rotation.vi"("Roll-Pitch-Yaw"=w619, "Input Position"=w618, "Mode"=T9."To User Coordinates") -> ("Output Position"=w616:sgl[])  [unwired: 2 in, 1 out]
          }
        }
        n236 = for {
          tunnel: w609 -> [w627] mode=indexing
          shift-right: [w622] -> w606
          shift-left: "\nDem Pos " -> [w625]
          tunnel: w602 -> [w620] mode=indexing
          n237 = Unbundle By Name(w627) -> ("Channel Name"=w626:string)
          n238 = call "Split_Ch_name.vi"("Ch name"=w626) -> ("Low level"=w624:string)  [unwired: 2 out]
          n239 = Format Into String(format string="%s=%.1f, " ("Format String"), w624, w620) -> (resulting string=w621:string)  [unwired: 2 in, 1 out]
          n240 = Concatenate Strings(w625, w621) -> (w622:string)
        }
        n241 = Concatenate Strings(w607, w606, w600) -> (w605:string)
      }
      frame 19 {
        # "Add Achieved Position"
        n242 = local read "Position Output XYZ"() -> (w628:sgl[])
        n243 = case shown="\"Work in Tunnel Coordinates\"" w629 {
          tunnel: w631 -> [_ w645]
          tunnel: [w642 w644] -> w630
          tunnel: w628 -> [w642 w643]
          frame "Work in Tunnel Coordinates" {
          }
          frame "Work in Model Coordinates" {
            n244 = call "Coordinate_rotation.vi"("Roll-Pitch-Yaw"=w645, "Input Position"=w643, "Mode"=T9."To User Coordinates") -> ("Output Position"=w644:sgl[])  [unwired: 2 in, 1 out]
          }
        }
        n245 = for {
          tunnel: w638 -> [w657] mode=indexing
          shift-right: [w652] -> w635
          shift-left: "\nAchieved Pos " -> [w655]
          tunnel: w630 -> [w650] mode=indexing
          n246 = Unbundle By Name(w657) -> ("Channel Name"=w656:string)
          n247 = call "Split_Ch_name.vi"("Ch name"=w656) -> ("Low level"=w654:string)  [unwired: 2 out]
          n248 = Format Into String(format string="%s=%.1f, " ("Format String"), w654, w650) -> (resulting string=w651:string)  [unwired: 2 in, 1 out]
          n249 = Concatenate Strings(w655, w651) -> (w652:string)
        }
        n250 = case shown="\"Read traverse position\"" w633 {
          tunnel: ["When requesting a move." "When reading position." "When teaching position."] -> w632
          frame "Move traverse" {
          }
          frame "Read traverse position" {
          }
          frame "Teach Position" {
          }
        }
        n251 = Concatenate Strings(w636, w635, w632) -> (w634:string)
      }
    }
  }
  "Error String" <- w12
